vi "Untitled 1.vi"() -> ()   [LabVIEW 2016, in "Untitled Library 2.lvlib"]
uses:
  Untitled Library 2.lvlib
panel:
  in  "kP":dbl format="%#_13g"
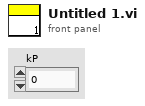
[diagram p1: front panel]
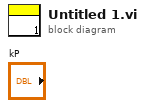
[diagram p0: block diagram]
diagram:
